vi "Draw Image at Position.vi"(7 "Image":T1, 9 "Top":i16, 10 "Left":i16, 11 "Picture In":picture) -> (3 "Picture":picture)   [LabVIEW 2020, in "TSnax UI.lvlib" / "TSnax UI Manager.lvclass"]
uses:
  TSnax UI Manager.lvclass
  TSnax UI Manager.lvclass/TSnax UI Manager.ctl
  Image.ctl
  TSnax UI.lvlib
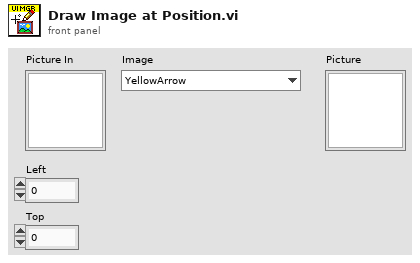
[diagram p1: front panel]
types:
  T1 = typedef "TSnax UI.lvlib/Image.ctl" = enum16{"YellowArrow", "GreenArrow"}
  T2 = typedef "imagedata.ctl" = cluster{"image type":i32, "image depth":i32, "image":u8[], "mask":u8[], "colors":u32[], "Rectangle":cluster{"left":i16, "top":i16, "right":i16, "bottom":i16}}
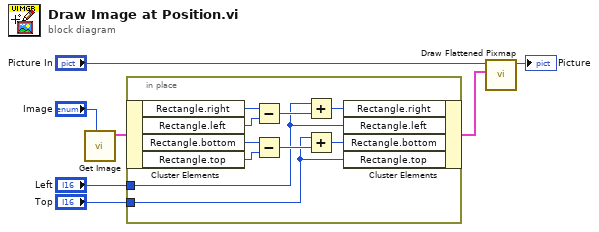
[diagram p0: block diagram]
diagram:
  n1 = call "Get Image.vi"("Image"="Image") -> ("Flattened Image"=w6:T2)  [unwired: 9 in, 1 out]
  n2 = in-place {
    in-place-border: "Left" -> [w9]
    in-place-border: "Top" -> [w8]
    n3 = in-place-cluster #1(w6) -> ("Rectangle.right"=w17:i16, "Rectangle.left"=w16:i16, "Rectangle.bottom"=w15:i16, "Rectangle.top"=w14:i16)
    n4 = Subtract(x=w17, y=w16) -> (x-y=w13:i16)
    n5 = Subtract(x=w15, y=w14) -> (x-y=w10:i16)
    n6 = Add(x=w9, y=w13) -> (x+y=w12:i16)
    n7 = Add(x=w8, y=w10) -> (x+y=w11:i16)
    n8 = in-place-cluster #1("Rectangle.right"=w12, "Rectangle.left"=w9, "Rectangle.bottom"=w11, "Rectangle.top"=w8) -> (w5:T2)
  }
  n9 = call <vilib>:"Draw Flattened Pixmap.vi"("image data"=w5, "picture"="Picture In") -> ("new picture"=→"Picture":picture)  [unwired: 7 in]
